vi "FPGA_target_read_memory.vi"(0 "addr_in":u32) -> (7 "data_mem0":u8, 9 "data_mem1":u32, 10 "next_addr_out":u32, 11 "data_mem2":u32, 13 "data_mem3":u32, 14 "addr_dup":u32)   [LabVIEW 2014]
doc: "Reads command data from memory specified by address."
uses:
  <vilib>/rvi/Memory/Memory_Emulation/nirvimemoryEmulation.vi
  <vilib>/rvi/Memory/Memory_Emulation/nirvimemoryFastEmulation.vi
  <vilib>/rvi/DataTransferAndStorage/Container/Common/niFpgaContainerGetUniqueNameForEmu.vi
  <vilib>/rvi/Memory/Memory_Emulation/niFpgaMemoryEmulationCacheClearOnFirstRun.vi
  <vilib>/rvi/Memory/Memory_Emulation/nirvimemoryEmulationManagerCache_MakeExclusive.vi
  <vilib>/rvi/Memory/Memory_Emulation/niFpgaMemoryEmulationValidateCache.vi
  <vilib>/rvi/Memory/Memory_Emulation/nirvimemoryEmulationManagerCache_InsertValue.vi
  <vilib>/Utility/error.llb/Clear Errors.vi
  <vilib>/rvi/Memory/Memory_Emulation/nirvimemoryEmulationManagerCache_ReleaseExclusive.vi
  <vilib>/rvi/Memory/Memory_Emulation/nirvimemoryEmulationManagerCache_GetValue.vi
  <vilib>/rvi/Emulation/niFpgaEmulationIsFPGAContextNoSignature.vi
  <vilib>/rvi/Emulation/niFpgaSctlEmulationGetInTimedLoop.vi
  <vilib>/rvi/Memory/Memory_Emulation/nirvimemoryEmulationManagerCache_SetValue.vi
  <vilib>/rvi/Emulation/niFpgaSctlEmulationResourceMgr.vi
  <vilib>/rvi/DataTransferAndStorage/Container/XNode/niFpgaContainer.xnode
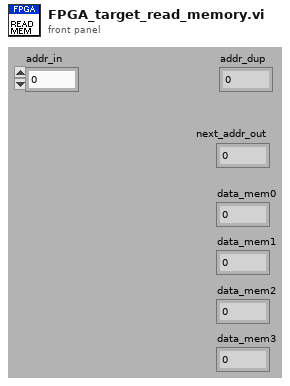
[diagram p1: front panel]
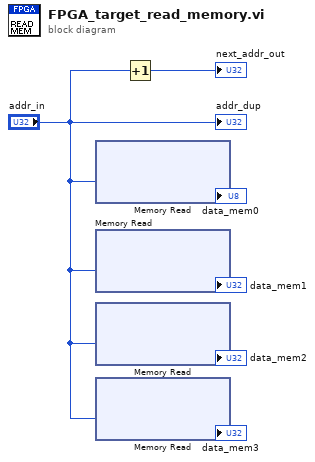
[diagram p0: block diagram]
diagram:
  n1 = xnode ("Memory Read")("Address"="addr_in") -> ("Data"=→"data_mem0":u8)  [unwired: 1 in, 1 out]
  n2 = xnode ("Memory Read")("Address"="addr_in") -> ("Data"=→"data_mem1":u32)  [unwired: 1 in, 1 out]
  n3 = xnode ("Memory Read")("Address"="addr_in") -> ("Data"=→"data_mem2":u32)  [unwired: 1 in, 1 out]
  n4 = xnode ("Memory Read")("Address"="addr_in") -> ("Data"=→"data_mem3":u32)  [unwired: 1 in, 1 out]
  n5 = Increment(x="addr_in") -> (x+1=→"next_addr_out":u32)
  "addr_dup" <- "addr_in"
